vi "PipBoy_GetIconsFromTdms.vi"() -> ()   [LabVIEW 2014]
panel:
  out "error out":errorcluster
  out "Array":picture[](array[picture])
  in  "Path":path
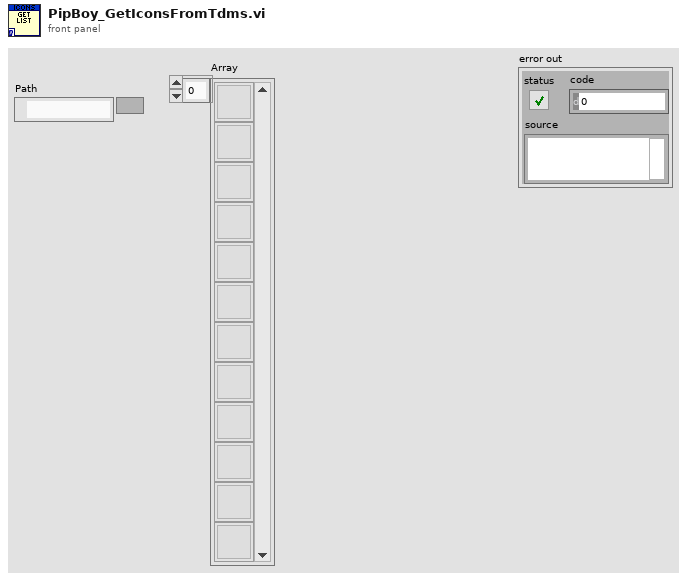
[diagram p1: front panel]
types:
  T1 = typedef "imagedata.ctl" = cluster{"image type":i32, "image depth":i32, "image":u8[], "mask":u8[], "colors":u32[], "Rectangle":cluster{"left":i16, "top":i16, "right":i16, "bottom":i16}}
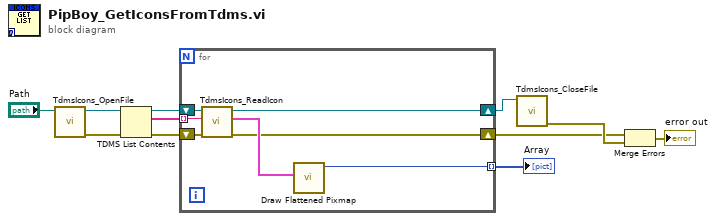
[diagram p0: block diagram]
diagram:
  n1 = call "TdmsIcons_OpenFile.vi"("Path"="Path") -> ("error out"=w9:errorcluster, "TdmsOut"=w10:refnum<k34>)  [unwired: 9 in]
  n2 = TDMS List Contents(4:w9, 7:w10) -> (0:w7:errorcluster, 2:w8:string[], 3:w6:refnum<k34>)  [unwired: 1 in, 1 out]
  n3 = for {
    tunnel: w8 -> [w15] mode=indexing
    shift-right: [w17] -> w5
    shift-left: w6 -> [w16]
    tunnel: [w13] -> w4 mode=indexing
    shift-right: [w12] -> w2
    shift-left: w7 -> [w18]
    n4 = call "TdmsIcons_ReadIcon.vi"("error in (no error)"=w18, "Function"=w15, "TdmsIn"=w16) -> ("error out"=w12:errorcluster, "Icon"=w14:T1, "TdmsOut"=w17:refnum<k34>)  [unwired: 6 in]
    n5 = call <vilib>:"Draw Flattened Pixmap.vi"("image data"=w14) -> ("new picture"=w13:picture)  [unwired: 8 in]
  }
  "Array" <- w4
  n6 = call "TdmsIcons_CloseFile.vi"("TdmsIn"=w5) -> ("error out"=w3:errorcluster)  [unwired: 9 in, 1 out]
  n7 = Merge Errors(w2, w3) -> (→"error out":errorcluster)
